vi "Init.vi"(8 "Project:Active Project":refnum<vi>, 9 "Application Instance":refnum<vi>, 10 "Name":string, 11 "First Library Script Strategy in":refnum<class "First Library Script Strategy.lvclass">) -> (3 "First Library Script Strategy out":refnum<class "First Library Script Strategy.lvclass">)   [LabVIEW 2021, in "_Create From Template.lvlib" / "Script Strategy.lvlib" / "First Library Script Strategy.lvclass"]
uses:
  First Library Script Strategy.lvclass
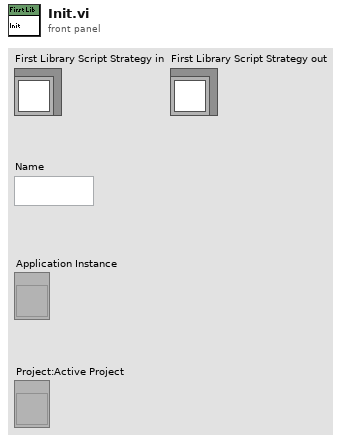
[diagram p1: front panel]
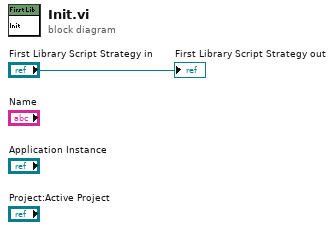
[diagram p0: block diagram]
diagram:
  "First Library Script Strategy out" <- "First Library Script Strategy in"
